vi "simpleLabVIEWRead.vi"() -> ()   [LabVIEW 2014]
uses:
  C:/MongoData/Drivers/mongo-csharp-driver-2.0.0-beta4/mongo-csharp-driver-2.0.0-beta4/src/MongoDB.Driver.Legacy/bin/Release/MongoDB.Driver.Legacy.dll
  MongoData/Drivers/mongo-csharp-driver-2.0.0-beta4/mongo-csharp-driver-2.0.0-beta4/src/MongoDB.Driver.Legacy/bin/Release/MongoDB.Driver.Legacy.dll
  C:/MongoData/Drivers/mongo-csharp-driver-2.0.0-beta4/mongo-csharp-driver-2.0.0-beta4/src/MongoDB.Driver.Legacy/bin/Release/MongoDB.Driver.dll
  MongoData/Drivers/mongo-csharp-driver-2.0.0-beta4/mongo-csharp-driver-2.0.0-beta4/src/MongoDB.Driver.Legacy/bin/Release/MongoDB.Driver.dll
  C:/MongoData/Drivers/mongo-csharp-driver-2.0.0-beta4/mongo-csharp-driver-2.0.0-beta4/src/MongoDB.Driver.Legacy/bin/Release/MongoDB.Bson.dll
  MongoData/Drivers/mongo-csharp-driver-2.0.0-beta4/mongo-csharp-driver-2.0.0-beta4/src/MongoDB.Driver.Legacy/bin/Release/MongoDB.Bson.dll
panel:
  out "ToString 2":string
  out "Count 2":i64
  in  "GetCollectionNames 3":refnum<k24>
  out "Count":i32
  in  "GetCollectionNames 2":refnum<k24>
  in  "GetCollectionNames":refnum<k24>
  out "ToString":string
  out "error out":errorcluster
  out "Array":string[](array[string])
  in  "MongoClientExtensions":refnum<k24>
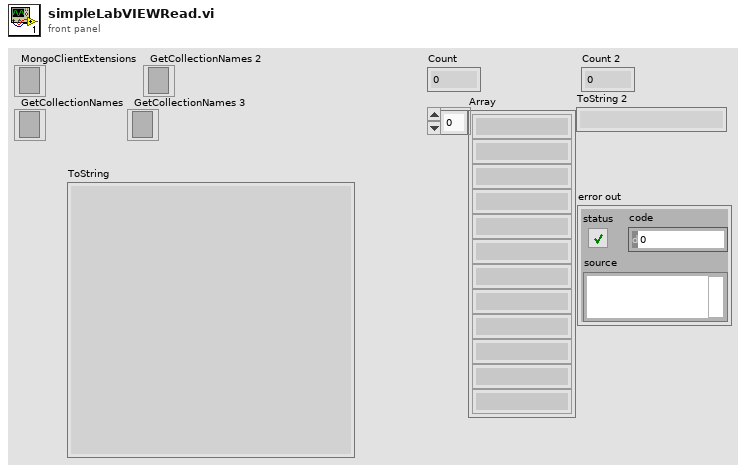
[diagram p1: front panel]
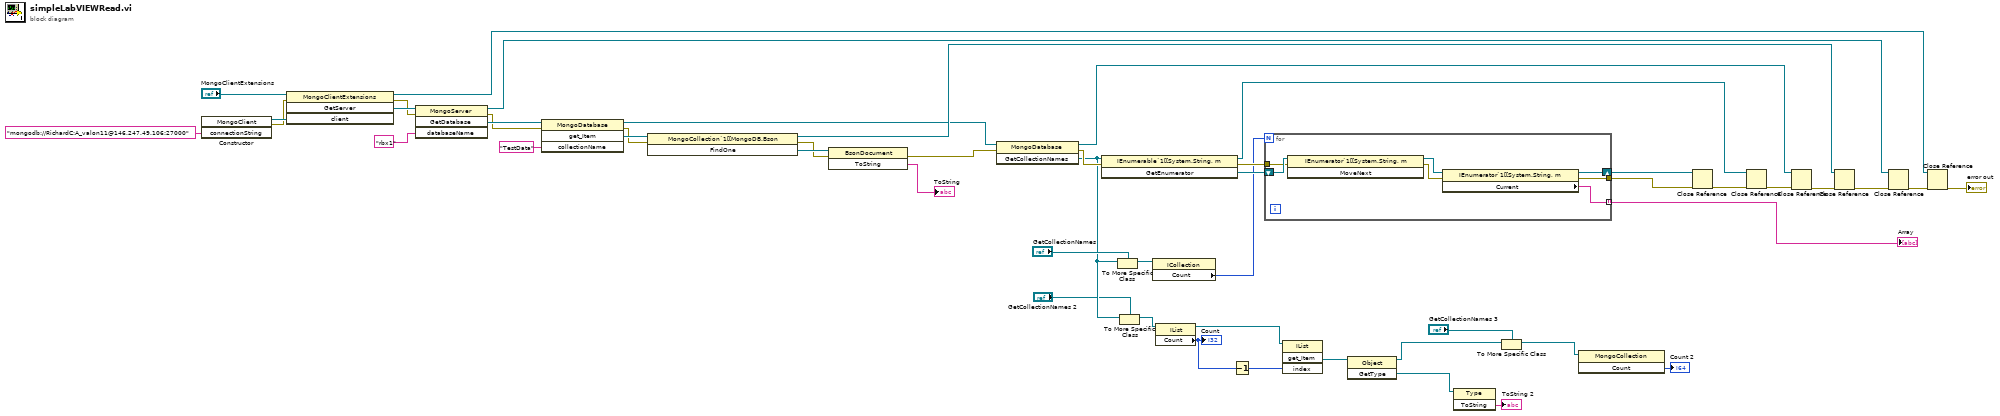
[diagram p0: block diagram]
diagram:
  n1 = constructor class="MongoClient"("connectionString"="mongodb://RichardC:A_valon11@146.247.49.106:27000") -> (reference out=w49:refnum<k24>, error out=w48:errorcluster)  [unwired: 3 in, 2 out]
  n2 = invoke class="MongoClientExtensions" method="GetServer"(reference="MongoClientExtensions", error in=w48, "client"=w49) -> (reference out=w44:refnum<k24>, error out=w45:errorcluster, "GetServer"=w46:refnum<k24>)  [unwired: 1 in, 1 out]
  n3 = invoke class="MongoServer" method="GetDatabase"(reference=w46, error in=w45, "databaseName"="rbx1") -> (reference out=w40:refnum<k24>, error out=w19:errorcluster, "GetDatabase"=w42:refnum<k24>)  [unwired: 1 in, 1 out]
  n4 = invoke class="MongoDatabase" method="get_Item"(reference=w42, error in=w19, "collectionName"="TestData") -> (reference out=w25:refnum<k24>, error out=w20:errorcluster, "get_Item"=w27:refnum<k24>)  [unwired: 1 in, 1 out]
  n5 = invoke class="MongoCollection`1[[MongoDB.Bson" method="FindOne"(reference=w27, error in=w20) -> (reference out=w26:refnum<k24>, error out=w22:errorcluster, "FindOne"=w23:refnum<k24>)  [unwired: 1 in]
  n6 = invoke class="BsonDocument" method="ToString"(reference=w23, error in=w22) -> (error out=w21:errorcluster, "ToString"=→"ToString":string)  [unwired: 1 in, 1 out]
  n7 = invoke class="MongoDatabase" method="GetCollectionNames"(reference=w25, error in=w21) -> (reference out=w24:refnum<k24>, error out=w39:errorcluster, "GetCollectionNames"=w13:refnum<k24>)  [unwired: 1 in]
  n8 = invoke class="IEnumerable`1[[System.String, m" method="GetEnumerator"(reference=w13, error in=w39) -> (reference out=w34:refnum<k24>, error out=w38:errorcluster, "GetEnumerator"=w17:refnum<k24>)  [unwired: 1 in]
  n9 = To More Specific Class(target class="GetCollectionNames", reference=w13) -> (specific class reference=w15:refnum<k24>)  [unwired: 1 in, 1 out]
  n10 = To More Specific Class(target class="GetCollectionNames 2", reference=w13) -> (specific class reference=w11:refnum<k24>)  [unwired: 1 in, 1 out]
  n11 = property class="ICollection"(reference=w15) -> ("Count"=w14:i32)  [unwired: 1 in, 2 out]
  n12 = property class="IList"(reference=w11) -> (reference out=w10:refnum<k24>, "Count"=w9:i32)  [unwired: 1 in, 1 out]
  "Count" <- w9
  n13 = Decrement(x=w9) -> (x-1=w7:i32)
  n14 = for {
    N: w14 -> [_]
    tunnel: w38 -> [w52]
    shift-right: [w56] -> w36
    shift-left: w17 -> [w54]
    tunnel: [w57] -> w37 mode=indexing
    tunnel: [w55] -> w35
    n15 = invoke class="IEnumerator`1[[System.String, m" method="MoveNext"(reference=w54, error in=w52) -> (reference out=w53:refnum<k24>, error out=w51:errorcluster)  [unwired: 1 in, 1 out]
    n16 = property class="IEnumerator`1[[System.String, m"(reference=w53, error in=w51) -> (reference out=w56:refnum<k24>, error out=w55:errorcluster, "Current"=w57:string)
  }
  "Array" <- w37
  n17 = invoke class="IList" method="get_Item"(reference=w10, "index"=w7) -> ("get_Item"=w8:refnum<k24>)  [unwired: 2 in, 3 out]
  n18 = invoke class="Object" method="GetType"(reference=w8) -> (reference out=w5:refnum<k24>, "GetType"=w2:refnum<k24>)  [unwired: 2 in, 1 out]
  n19 = invoke class="Type" method="ToString"(reference=w2) -> ("ToString"=→"ToString 2":string)  [unwired: 2 in, 2 out]
  n20 = To More Specific Class(target class="GetCollectionNames 3", reference=w5) -> (specific class reference=w4:refnum<k24>)  [unwired: 1 in, 1 out]
  n21 = invoke class="MongoCollection" method="Count"(reference=w4) -> ("Count"=→"Count 2":i64)  [unwired: 2 in, 2 out]
  n22 = Close Reference(reference=w36, error in (no error)=w35) -> (error out=w33:errorcluster)
  n23 = Close Reference(reference=w34, error in (no error)=w33) -> (error out=w32:errorcluster)
  n24 = Close Reference(reference=w24, error in (no error)=w32) -> (error out=w31:errorcluster)
  n25 = Close Reference(reference=w26, error in (no error)=w31) -> (error out=w29:errorcluster)
  n26 = Close Reference(reference=w40, error in (no error)=w29) -> (error out=w28:errorcluster)
  n27 = Close Reference(reference=w44, error in (no error)=w28) -> (error out=→"error out":errorcluster)
